vi "raptor_build_enface.vi"(4 "Track Surface":bool, 7 "Depth":i64, 8 "error in (no error)":errorcluster, 9 "Volume En Face In":T2, 10 "Build Record":T1[](array[typedef]), 11 "B Scans":T2[](array[typedef])) -> (0 "error out":errorcluster, 3 "Volume En Face Out":T2)   [LabVIEW 2016]
uses:
  <vilib>/vision/Image Controls.llb/IMAQ Image.ctl
  typedef/build_record.ctl
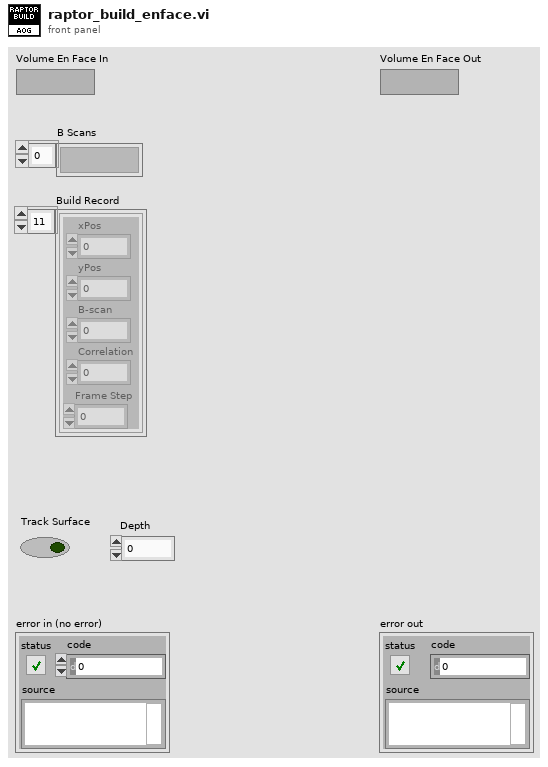
[diagram p1: front panel]
types:
  T1 = typedef "build_record.ctl" = cluster{"xPos":i32, "yPos":i32, "B-scan":i32, "Correlation":dbl, "Frame Step":dbl}
  T2 = typedef "IMAQ Image.ctl" = refnum<image>
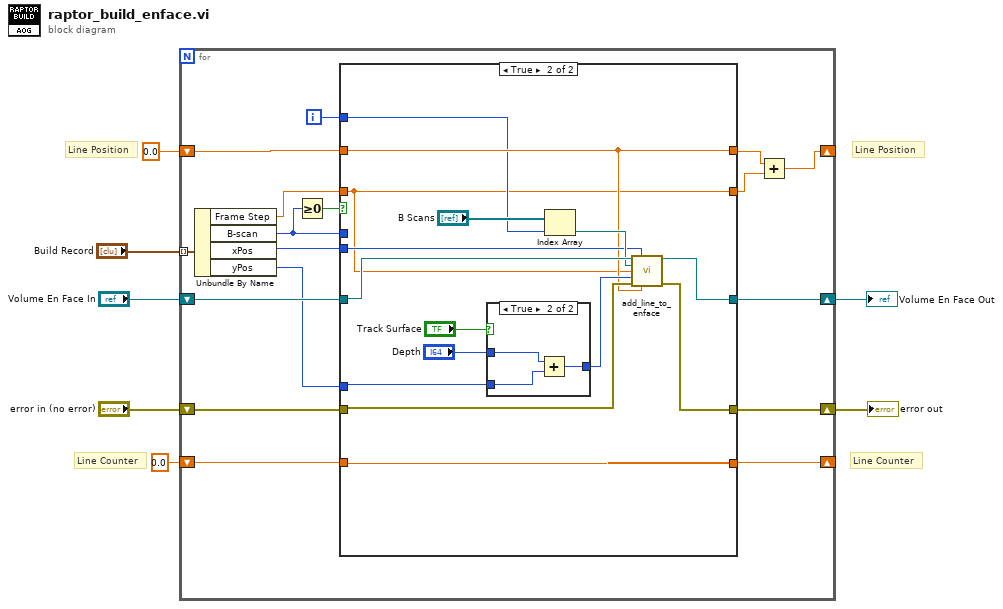
[diagram p0: block diagram]
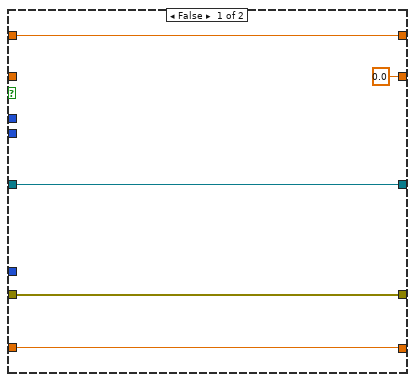
[diagram p2: hidden frame]
diagram:
  # "Line Position"
  # "Line Position"
  # "Line Counter"
  # "Line Counter"
  n1 = for {
    tunnel: "Build Record" -> [w23] mode=indexing
    shift-right: [w21] -> w7
    shift-left: "Volume En Face In" -> [w24]
    shift-right: [w19] -> w6
    shift-left: "error in (no error)" -> [w20]
    shift-right: [w17] -> _
    shift-left: 0.0 -> [w18]
    shift-right: [w8] -> _
    shift-left: 0.0 -> [w11]
    i -> [w12]
    n2 = Unbundle By Name(w23) -> ("Frame Step"=w13:dbl, "B-scan"=w16:i32, "xPos"=w22:i32, "yPos"=w14:i32)
    n3 = Greater Or Equal To 0?(x=w16) -> (x >= 0?=w15:bool)
    n4 = case shown="True" w15 {
      tunnel: w24 -> [w27 w44]
      tunnel: w16 -> [_ _]
      tunnel: w22 -> [_ w33]
      tunnel: [w27 w41] -> w21
      tunnel: w20 -> [w28 w40]
      tunnel: [w28 w39] -> w19
      tunnel: w18 -> [w29 w34]
      tunnel: [w29 w34] -> w17
      tunnel: w14 -> [_ w35]
      tunnel: w11 -> [w26 w32]
      tunnel: [w26 w32] -> w9
      tunnel: w13 -> [_ w30]
      tunnel: w12 -> [_ w31]
      tunnel: [0.0 ("Frame Step") w30] -> w10
      frame False {
      }
      frame True {
        n5 = case shown="True" "Track Surface" {
          tunnel: "Depth" -> [w45 w48]
          tunnel: w35 -> [_ w47]
          tunnel: [w45 w46] -> w36
          frame False {
          }
          frame True {
            n6 = Add(x=w48, y=w47) -> (x+y=w46:i64)
          }
        }
        n7 = Index Array(array="B Scans", index=w31) -> (element=w42:T2)
        n8 = call "add_line_to_enface.vi"("En Face Image"=w44, "Shift"=w33, "Raw Image"=w42, "Add Height"=w30, "Input Line"=w36, "error in (no error)"=w40, "Output Line"=w32) -> ("En Face Image Out"=w41:T2, "error out"=w39:errorcluster)  [unwired: 7 in]
      }
    }
    n9 = Add(x=w9, y=w10) -> (x+y=w8:dbl)
  }
  "error out" <- w6
  "Volume En Face Out" <- w7
